vi "cw_6_4.vi"() -> ()   [LabVIEW 2022 SP3]
panel:
  out "Users 4":string
  out "Users 3":string
  out "Users 2":string
  out "Users":string
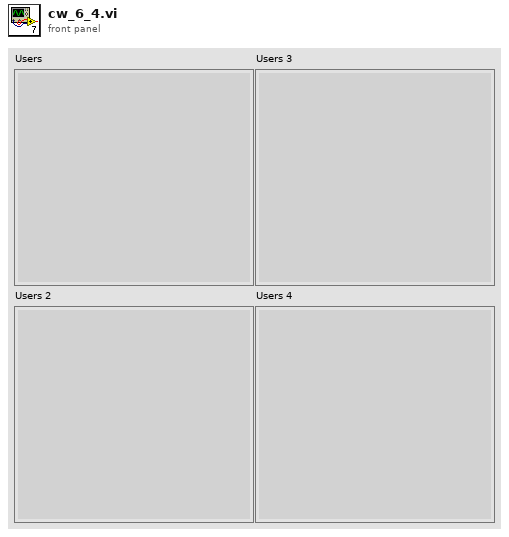
[diagram p1: front panel]
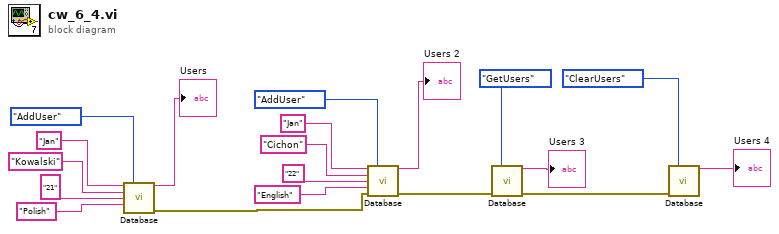
[diagram p0: block diagram]
diagram:
  n1 = call "Database.vi"("Name"="Jan", "Action"=enum16{"ClearUsers", "GetUsers", "AddUser"}."AddUser", "Surname"="Kowalski", "Age"="21", "Nationality"="Polish") -> ("Users"=→"Users":string, "error constant"=w7:errorcluster)  [unwired: 9 in]
  n2 = call "Database.vi"("Name"="Jan", "Action"=enum16{"ClearUsers", "GetUsers", "AddUser"}."AddUser", "Surname"="Cichon", "Age"="22", "Nationality"="English", "error in"=w7) -> ("Users"=→"Users 2":string, "error constant"=w4:errorcluster)  [unwired: 8 in]
  n3 = call "Database.vi"("Action"=enum16{"ClearUsers", "GetUsers", "AddUser"}."GetUsers", "error in"=w4) -> ("Users"=→"Users 3":string, "error constant"=w1:errorcluster)  [unwired: 12 in]
  n4 = call "Database.vi"("Action"=enum16{"ClearUsers", "GetUsers", "AddUser"}."ClearUsers", "error in"=w1) -> ("Users"=→"Users 4":string)  [unwired: 12 in, 1 out]
